vi "RPC Get Relative Path.vi"(2 "Base Path (empty)":path, 3 "Absolute Path (empty)":path) -> (0 "Path Relative to Base":path)   [LabVIEW 2011]
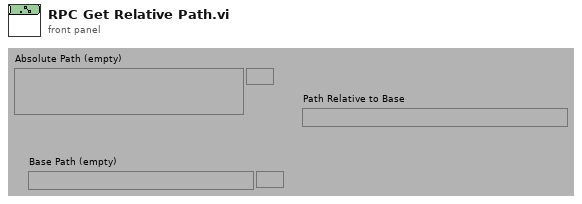
[diagram p1: front panel]
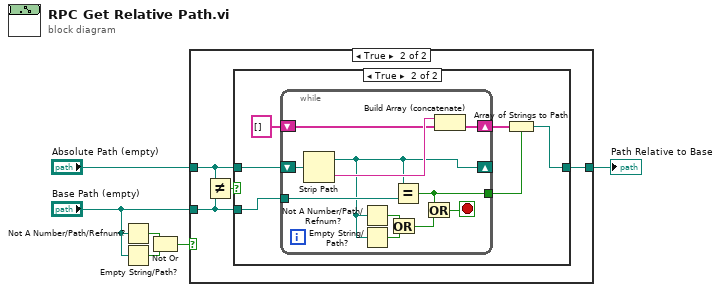
[diagram p0: block diagram]
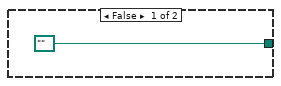
[diagram p3: hidden frame]
diagram:
  n1 = Not A Number/Path/Refnum?(number/path/refnum="Base Path (empty)") -> (NaN/Path/Refnum?=w3:bool)
  n2 = Empty String/Path?(string/path="Base Path (empty)") -> (empty?=w4:bool)
  n3 = Not Or(1:w4, 2:w3) -> (0:w1:bool)
  n4 = case shown="True" w1 {
    tunnel: "Base Path (empty)" -> [_ w10]
    tunnel: "Absolute Path (empty)" -> [w7 w11]
    tunnel: [w7 w8] -> w5
    frame False {
    }
    frame True {
      n5 = Not Equal?(x=w11, y=w10) -> (x != y?=w9:bool)
      n6 = case shown="True" w9 {
        tunnel: w11 -> [_ w17]
        tunnel: w10 -> [_ w18]
        tunnel: [path "" w14] -> w8
        frame False {
        }
        frame True {
          n7 = while {
            tunnel: w18 -> [w29]
            shift-right: [w25] -> w15
            shift-left: string[] [] -> [w24]
            shift-right: [w19] -> _
            shift-left: w17 -> [w27]
            tunnel: [w23] -> w13
            stop <- w28 stop-if-true
            n8 = Strip Path(path=w27) -> (stripped path=w19:path, name=w26:string)
            n9 = Not A Number/Path/Refnum?(number/path/refnum=w19) -> (NaN/Path/Refnum?=w22:bool)
            n10 = Empty String/Path?(string/path=w19) -> (empty?=w21:bool)
            n11 = Or(x=w22, y=w21) -> (x .or. y?=w20:bool)
            n12 = Equal?(x=w19, y=w29) -> (x = y?=w23:bool)
            n13 = Or(x=w23, y=w20) -> (x .or. y?=w28:bool)
            n14 = Build Array (concatenate)(w26, w24) -> (w25:string[])
          }
          n15 = Array of Strings to Path(0:w15, 1:w13) -> (2:w14:path)
        }
      }
    }
  }
  "Path Relative to Base" <- w5
